vi "Preview Stack.vi"(8 "error in (no error)":errorcluster, 10 "Stack Preview":dbl[](array[numeric]), 11 "UPNCalculatorGUI in":refnum<class "UPNCalculatorGUI.lvclass">) -> (0 "error out":errorcluster, 3 "UPNCalculatorGUI out":refnum<class "UPNCalculatorGUI.lvclass">)   [LabVIEW 2012, in "UPNCalculatorGUI Actor.lvlib" / "UPNCalculatorGUI.lvclass"]
doc: "This VI set Stack values on a Frontpanel via property node."
uses:
  UPNCalculatorGUI.lvclass
  UPNCalculatorGUI.lvclass/UPNCalculatorGUI.ctl
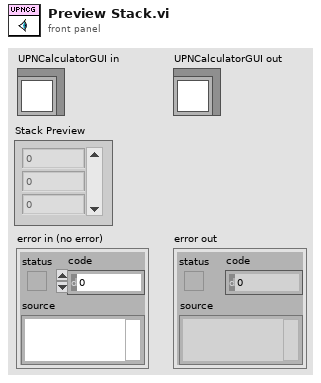
[diagram p1: front panel]
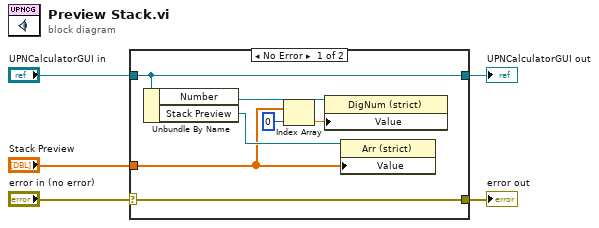
[diagram p0: block diagram]
diagram:
  n1 = case shown="No Error" "error in (no error)" {
    selector: "error in (no error)" -> [w12 w14]
    tunnel: [w12 w14] -> w4
    tunnel: [w11 w13] -> w2
    tunnel: "UPNCalculatorGUI in" -> [w11 w13]
    tunnel: "Stack Preview" -> [w7 _]
    frame No Error {
      n2 = Unbundle By Name(w11) -> ("Number"=w10:refnum<vi>, "Stack Preview"=w9:refnum<vi>)
      n3 = Index Array(array=w7, index=0) -> (element=w8:dbl)
      n4 = property class="DigNum (strict)"(reference=w10, "Value"=w8) -> ()  [unwired: 1 in, 2 out]
      n5 = property class="Arr (strict)"(reference=w9, "Value"=w7) -> ()  [unwired: 1 in, 2 out]
    }
    frame Error {
    }
  }
  "error out" <- w4
  "UPNCalculatorGUI out" <- w2
